vi "Feather Plot.vi"() -> ()   [LabVIEW 2020]
doc: "This VI shows how to use the 2D Feather Plot."
uses:
  <vilib>/Math Plots/2D Math Plots/2D Feather/2D Feather XCtrl/2D Feather.xctl
  <vilib>/Math Plots/2D Math Plots/2D Feather/2D Feather Datatype/Public/Plot Helper (Vector).vi
  <vilib>/Math Plots/2D Math Plots/2D Feather/2D Feather Datatype/2D Feather Datatype.lvclass
panel:
  out "Feather Plot":refnum<class "2D Plot Datatype.lvclass">[](xcontrol)
  # "Overview: Demonstrates the Feather Plot indicator.\nInstructions:\nRun the VI."
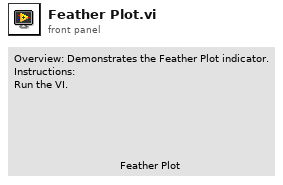
[diagram p1: front panel]
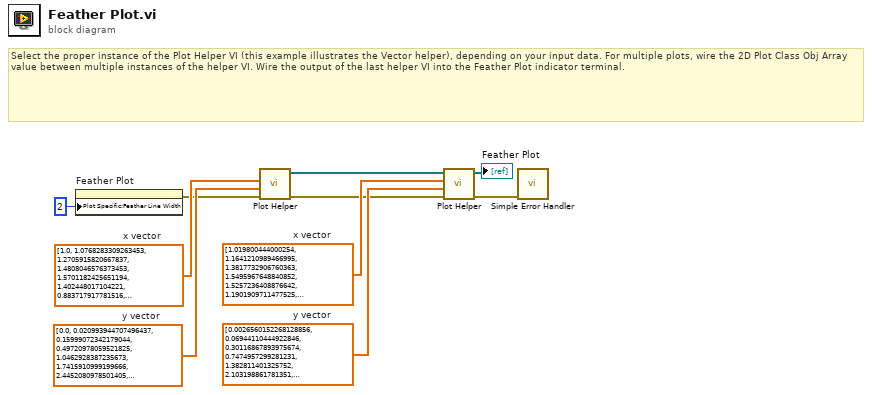
[diagram p0: block diagram]
diagram:
  w6 = dbl[] [0.0026560152268128856, 0.06944110444922846, 0.30116867893975674, 0.7474957299281231, 1.382811401325752, 2.103198861781351, 2.7434121305807273, 3.111097497861204, 3.031572752743336, 2.3938194143320635, 1.1875196772173493, -0.47778937973221614, -2.3772352019792695, -4.200106017646215, -5.60061537767341, -6.261650404361444]  # y vector
  w7 = dbl[] [1.019800444000254, 1.1641210989466995, 1.3817732906760363, 1.5495967648840852, 1.5257236408876642, 1.1901909711477525, 0.48341481336685965, -0.5666324724208438, -1.8356379394706885, -3.11602769749675, -4.15087906547777, -4.683131143648991, -4.510959187852466, -3.5382353568596963, -1.8091731236584692, 0.48138779955473987]  # x vector
  w8 = dbl[] [0.0, 0.020993944707496437, 0.15999072342179044, 0.49720978059521825, 1.0462928387235673, 1.7415910999199666, 2.4452080978501405, 2.973210704028148, 3.13616913911563, 2.785809855508077, 1.8577719881465196, 0.4006625540155292, -1.4161597293451875, -3.319741346482114, -4.974435557529722, -6.040437218101122]  # y vector
  w9 = dbl[] [1.0, 1.0768283309263453, 1.2705915820667837, 1.4808046576373453, 1.5701182425651194, 1.402448017104221, 0.883717917781516, -0.004255520232125165, -1.1850920347630094, -2.489832012195616, -3.6808536020953246, -4.49438199509229, -4.694091138972588, -4.125447538444419, -2.759527293574747, -0.7163227025431892]  # x vector
  # "Select the proper instance of the Plot Helper VI (this example illustrates the Vector helper), depending on your input data. For multiple plots, wire the 2D Plot Class Obj Array value between multiple instances of the helper VI. Wire the output of the last helper VI into the Feather Plot indicator terminal."
  n1 = property on="Feather Plot" class="2D Feather (strict)"("Plot Specific:Feather Line Width"=u8 2) -> (error out=w2:errorcluster)  [unwired: 2 in, 1 out]
  n2 = call-poly <vilib>:"Plot Helper.vi"("error in (no error)"=w2, "y vector"=w8, "x vector"=w9) -> ("error out"=w3:errorcluster, "2D Plot Class Obj Array out"=w10:refnum<class "2D Plot Datatype.lvclass">[])  [unwired: 1 in, 6 out]
  n3 = call-poly <vilib>:"Plot Helper.vi"("error in (no error)"=w3, "y vector"=w6, "x vector"=w7, "2D Plot Class Obj Array in"=w10) -> ("error out"=w4:errorcluster, "2D Plot Class Obj Array out"=→"Feather Plot":refnum<class "2D Plot Datatype.lvclass">[])  [unwired: 6 out]
  n4 = call <vilib>:"Simple Error Handler.vi"("error in (no error)"=w4) -> ()  [unwired: 4 in, 5 out]
